vi "Copy Built Directory Up Two Levels.vi"(5 "Files Generated by Build":path[](array[path]), 6 "Top Level/Always Included VIs":path[](array[path]), 7 "Destination Path":path, 8 "error in (no error)":errorcluster, 9 "Target Name":string, 10 "Build Specification Name":string, 11 "Project Path":path) -> (0 "error out":errorcluster)   [LabVIEW 2017]
doc: "This VI is called after each run of a build specification. The VI will copy the generated LLB (Engine or System Explorer) into the VeriStand Custom Device folder (...\\Documents\\National Instruments\\NI VeriStand 2013...)."
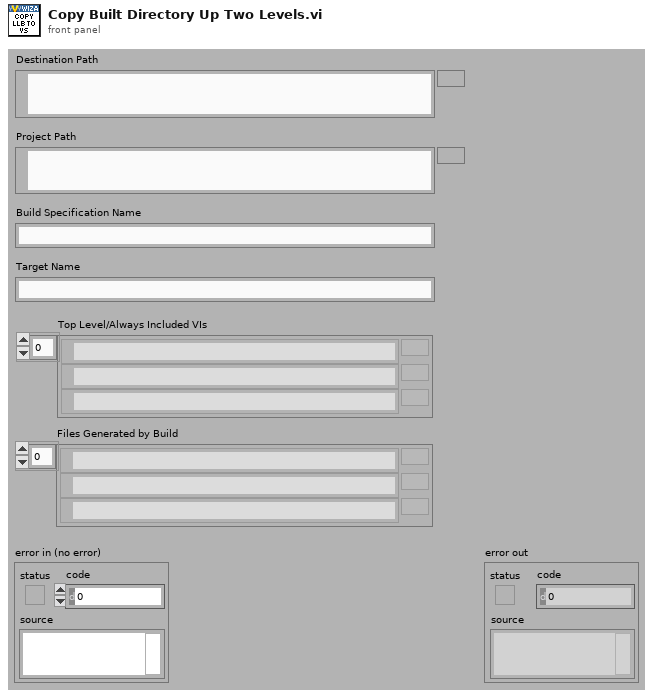
[diagram p1: front panel]
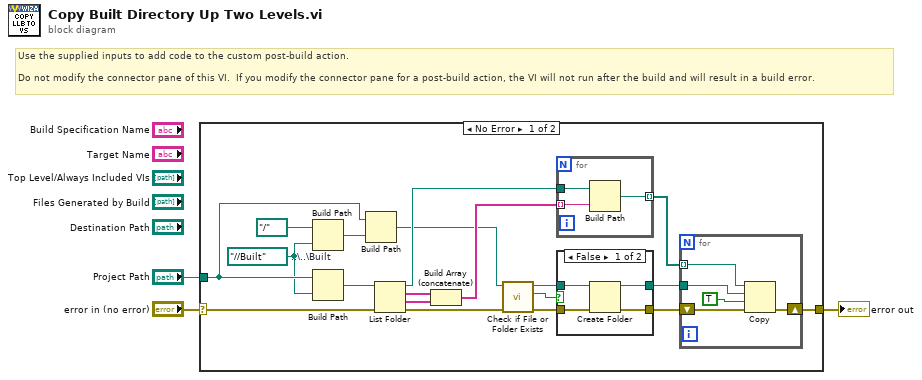
[diagram p0: block diagram]
diagram:
  # "Use the supplied inputs to add code to the custom post-build action.\n\nDo not modify the connector pane of this VI.  If you modify the connector pane for a post-build action, the VI will not run after the build and will result in a build error."
  n1 = case shown="No Error" "error in (no error)" {
    selector: "error in (no error)" -> [w14 w37]
    tunnel: [w15 w37] -> w1
    tunnel: "Project Path" -> [w7 _]
    frame No Error {
      w4 = path "../../Built"  # ..\..\Built
      n2 = Build Path(base path=path "../..", name or relative path=w4) -> (appended path=w8:path)
      n3 = Build Path(base path=w7, name or relative path=w4) -> (appended path=w16:path)
      n4 = Build Path(base path=w7, name or relative path=w8) -> (appended path=w6:path)
      n5 = List Folder(path=w16, error in=w14) -> (path out=w19:path, filenames=w11:string[], folder names=w10:string[], error out=w17:errorcluster)  [unwired: 2 in]
      n6 = Build Array (concatenate)(w11, w10) -> (w9:string[])
      n7 = call <vilib>:"Check if File or Folder Exists.vi"("error in (no error)"=w17, "path"=w6) -> ("error out"=w20:errorcluster, "file or folder exists?"=w22:bool, "dup path"=w21:path)  [unwired: 7 in]
      n8 = for {
        tunnel: w9 -> [w35] mode=indexing
        tunnel: w19 -> [w36]
        tunnel: [w34] -> w18 mode=indexing
        n9 = Build Path(base path=w36, name or relative path=w35) -> (appended path=w34:path)
      }
      n10 = case shown="False" w22 {
        tunnel: w21 -> [w26 w28]
        tunnel: w20 -> [w25 w27]
        tunnel: [w24 w28] -> w13
        tunnel: [w23 w27] -> w12
        frame False {
          n11 = Create Folder(path (use dialog)=w26, error in=w25) -> (created path=w24:path, error out=w23:errorcluster)  [unwired: 1 in, 1 out]
        }
        frame True {
        }
      }
      n12 = for {
        tunnel: w18 -> [w30] mode=indexing
        shift-right: [w31] -> w15
        shift-left: w12 -> [w32]
        tunnel: w13 -> [w29]
        n13 = Copy(8:w32, 9:TRUE ("overwrite (F)"), 10:w29, 11:w30) -> (0:w31:errorcluster)  [unwired: 1 in, 2 out]
      }
    }
    frame Error {
    }
  }
  "error out" <- w1
